vi "m10.wf.append2.vi"(4 "error in (no error)":errorcluster, 6 "Waveform In 2":waveform(dbl), 7 "Waveform In":waveform(dbl)) -> (0 "error out":errorcluster, 3 "Waveform Out":waveform(dbl))   [LabVIEW 2009]
uses:
  <vilib>/Waveform/WDTOps.llb/WDT Append Waveforms DBL.vi
  <vilib>/Waveform/WDTOps.llb/WDT Number of Waveform Samples DBL.vi
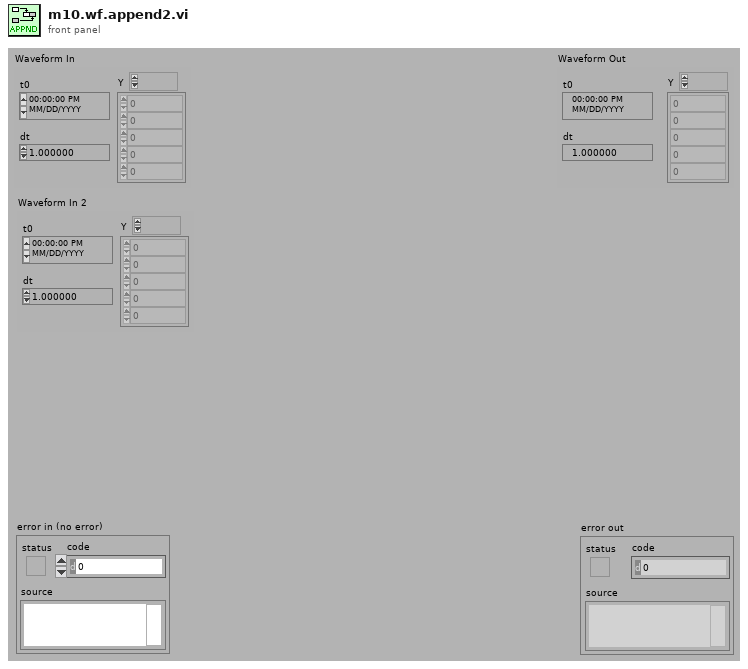
[diagram p1: front panel]
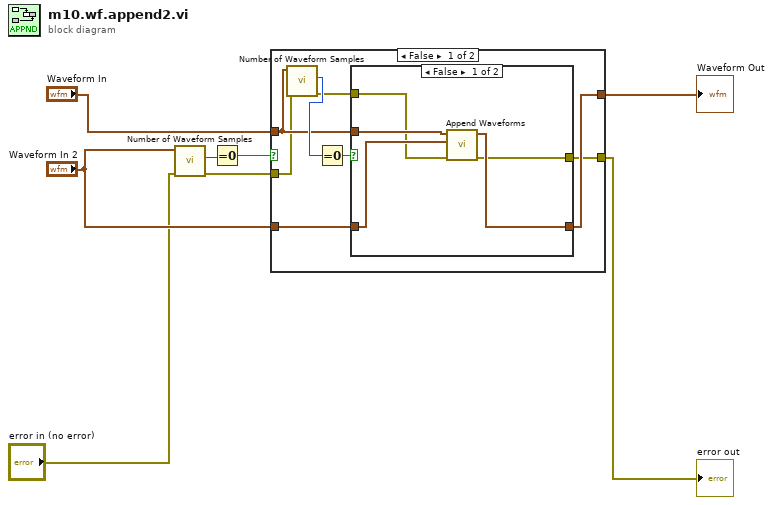
[diagram p0: block diagram]
diagram:
  n1 = call-poly <vilib>:"Number of Waveform Samples.vi"("error in (no error)"="error in (no error)", "waveform in"="Waveform In 2") -> ("error out"=w2:errorcluster, "number of samples"=w8:i32)  [unwired: 7 in, 1 out]
  n2 = Equal To 0?(x=w8) -> (x = 0?=w7:bool)
  n3 = case shown="False" w7 {
    tunnel: "Waveform In" -> [w12 w25]
    tunnel: "Waveform In 2" -> [w14 _]
    tunnel: [w13 w25] -> w4
    tunnel: w2 -> [w11 w24]
    tunnel: [w9 w24] -> w1
    frame #0 {
      n4 = call-poly <vilib>:"Number of Waveform Samples.vi"("error in (no error)"=w11, "waveform in"=w12) -> ("error out"=w10:errorcluster, "number of samples"=w16:i32)  [unwired: 7 in, 1 out]
      n5 = Equal To 0?(x=w16) -> (x = 0?=w15:bool)
      n6 = case shown="False" w15 {
        tunnel: [w19 w23] -> w13
        tunnel: w14 -> [w20 w23]
        tunnel: w12 -> [w21 _]
        tunnel: w10 -> [w18 w22]
        tunnel: [w17 w22] -> w9
        frame #0 {
          n7 = call-poly <vilib>:"Append Waveforms.vi"("error in (no error)"=w18, "waveform B"=w20, "waveform A"=w21) -> ("error out"=w17:errorcluster, "waveform out"=w19:waveform(dbl))  [unwired: 7 in]
        }
        frame #1 {
        }
      }
    }
    frame #1 {
    }
  }
  "Waveform Out" <- w4
  "error out" <- w1
